vi "configTrigger.vi"(2 "error in (no error)":errorcluster, 3 "IMAQ Session In":refnum<k11>) -> (0 "error out":errorcluster, 1 "IMAQ Session Out":refnum<k11>)   [LabVIEW 2017]
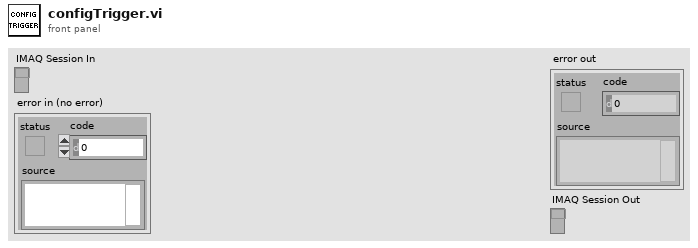
[diagram p1: front panel]
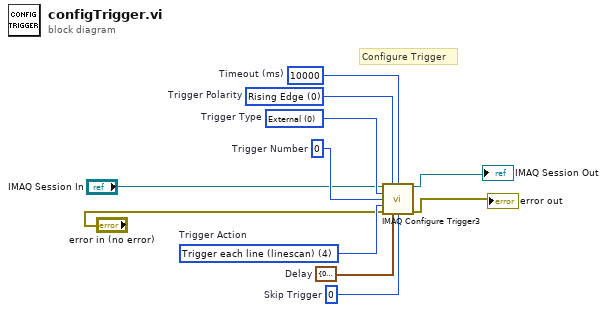
[diagram p0: block diagram]
diagram:
  w5 = cluster{"Value":dbl, "Units":u32} {"Value"=0.0, "Units"=5}  # Delay
  w8 = u32 10000  # Timeout (ms)
  w9 = u32 0 items=["Rising Edge", "Falling Edge"]  # Trigger Polarity
  w11 = u32 0  # Skip Trigger
  w6 = u32 4 items=["Disabled", "Trigger start of acquisition", "Trigger start of each buffer list", "Trigger each buffer", "Trigger each line (linescan)", "Trigger end of acquisition"]  # Trigger Action
  w7 = u32 0  # Trigger Number
  w10 = u32 0 items=["External"=0, "RTSI"=1, "ISO In"=2, "Scaled Encoder"=5]  # Trigger Type
  # "Configure Trigger"
  n1 = call <vilib>:"IMAQ Configure Trigger3.vi"("IMAQ Session In"="IMAQ Session In", "Polarity"=w9, "Frame timeout (ms)"=w8, "Type"=w10, "Line Number"=w7, "Action"=w6, "error in (no error)"="error in (no error)", "Delay"=w5, "Skip trigger (linescan only)"=w11) -> ("IMAQ Session Out"=→"IMAQ Session Out":refnum<k11>, "error out"=→"error out":errorcluster)  [unwired: 5 out]
